vi "EnableCell.vi"(0 "MenuCol in":refnum<class "MenuCol.lvclass">, 1 "Col Array Ref in":refnum<vi>, 5 "Cell Position":T1, 7 "Table Data in":string[][](array[string]), 9 "Table CtlRef In":refnum<vi>, 11 "error in (no error)":errorcluster) -> (4 "MenuCol out":refnum<class "MenuCol.lvclass">, 8 "Table Data out":string[][](array[string]), 10 "Table CtlRef Out":refnum<vi>, 14 "Needs 2nd pass":bool, 15 "error out":errorcluster)   [LabVIEW 2013, in "MenuCol.lvclass"]
uses:
  MenuCol.lvclass
  <vilib>/Utility/miscctls.llb/LVRowAndColumnTypeDef.ctl
  Column/Column.lvclass/Column.ctl
  Column/Column.lvclass
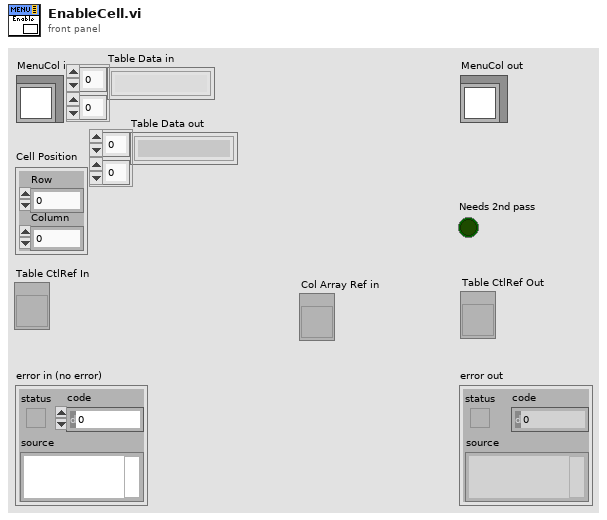
[diagram p1: front panel]
types:
  T1 = typedef "LVRowAndColumnTypeDef.ctl" = cluster{"Row":i32, "Column":i32}
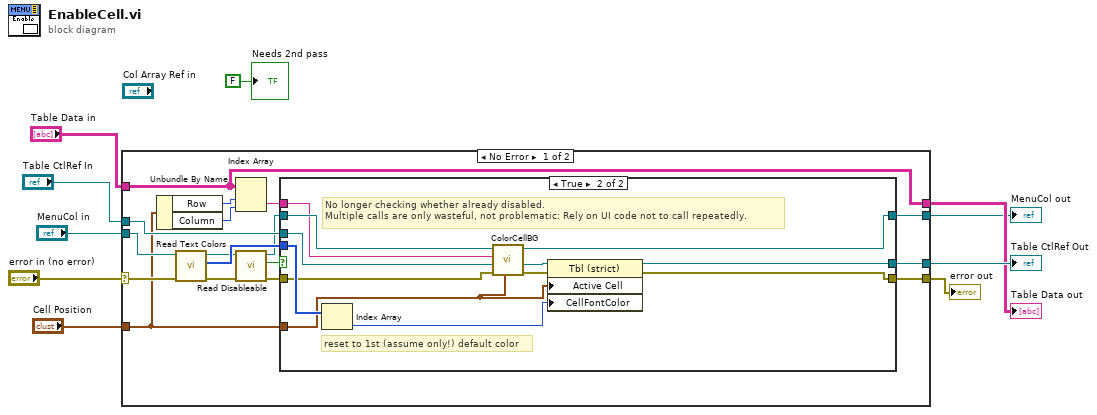
[diagram p0: block diagram]
diagram:
  n1 = case shown="No Error" "error in (no error)" {
    selector: "error in (no error)" -> [w18 w46]
    tunnel: [w25 w46] -> w4
    tunnel: [w22 w45] -> w1
    tunnel: "MenuCol in" -> [w20 w45]
    tunnel: "Cell Position" -> [w15 _]
    tunnel: "Table CtlRef In" -> [w27 w44]
    tunnel: [w26 w44] -> w3
    tunnel: "Table Data in" -> [w11 w43]
    tunnel: [w11 w43] -> w2
    frame No Error {
      n2 = Unbundle By Name(w15) -> ("Row"=w14:i32, "Column"=w13:i32)
      n3 = call "Read Text Colors.vi"("error in (no error)"=w18, "Column in"=w20) -> ("error out"=w16:errorcluster, "Text Colors"=w24:u32[], "Column out"=w19:refnum<class "MenuCol.lvclass">)  [unwired: 7 in]
      n4 = Index Array(array=w11, index (row)=w14, index (col)=w13) -> (element=w12:string)
      n5 = call "Read Disableable.vi"("error in (no error)"=w16, "Column in"=w19) -> ("error out"=w17:errorcluster, "Disableable?"=w23:bool, "Column out"=w21:refnum<class "MenuCol.lvclass">)  [unwired: 7 in]
      n6 = case shown="True" w23 {
        tunnel: w27 -> [w30 w36]
        tunnel: [w30 w42] -> w26
        tunnel: w15 -> [_ w38]
        tunnel: w17 -> [w29 w37]
        tunnel: [w29 w41] -> w25
        tunnel: w24 -> [_ w40]
        tunnel: w21 -> [w28 w33]
        tunnel: [w28 w32] -> w22
        tunnel: w12 -> [_ w31]
        frame False {
          # "Do nothing if column must always be enabled!"
        }
        frame True {
          # "reset to 1st (assume only!) default color"
          # "No longer checking whether already disabled. \nMultiple calls are only wasteful, not problematic: Rely on UI code not to call repeatedly."
          n7 = Index Array(array=w40) -> (element=w39:u32)  [unwired: 1 in]
          n8 = call-dynamic "ColorCellBG.vi"("Cell Position"=w38, "error in (no error)"=w37, "Table CtlRef In"=w36, "Value"=w31, "MenuCol in"=w33) -> ("error out"=w34:errorcluster, "Table CtlRef Out"=w35:refnum<vi>, "MenuCol out"=w32:refnum<class "MenuCol.lvclass">)  [unwired: 4 in]
          n9 = property class="Tbl (strict)"(reference=w35, error in=w34, "Active Cell"=w38, "CellFontColor"=w39) -> (reference out=w42:refnum<vi>, error out=w41:errorcluster)
        }
      }
    }
    frame Error {
    }
  }
  "error out" <- w4
  "MenuCol out" <- w1
  "Table CtlRef Out" <- w3
  "Table Data out" <- w2
  "Needs 2nd pass" <- FALSE ("Needs 2nd pass")
